vi "Leaderboard test 2.vi"() -> ()   [LabVIEW 2020, in "Visualisation.lvclass"]
uses:
  Visualisation.lvclass
  Application/Globals.vi
  Data Manager/Data Manager.lvclass
  Application/Application.lvlib
panel:
  out "Distance":T1(slide)={"Numeric"=0.0, "Numeric"=29.941887583444593, "Numeric"=34.779659813084116} scale=0.0..48.9661
  out "Leaderboard":T2(array[cluster]) {"Distance" scale=0.0..48.9661}
  out "B Total":dbl format="%0.1f km"
  out "A Total":dbl format="%0.1f km"
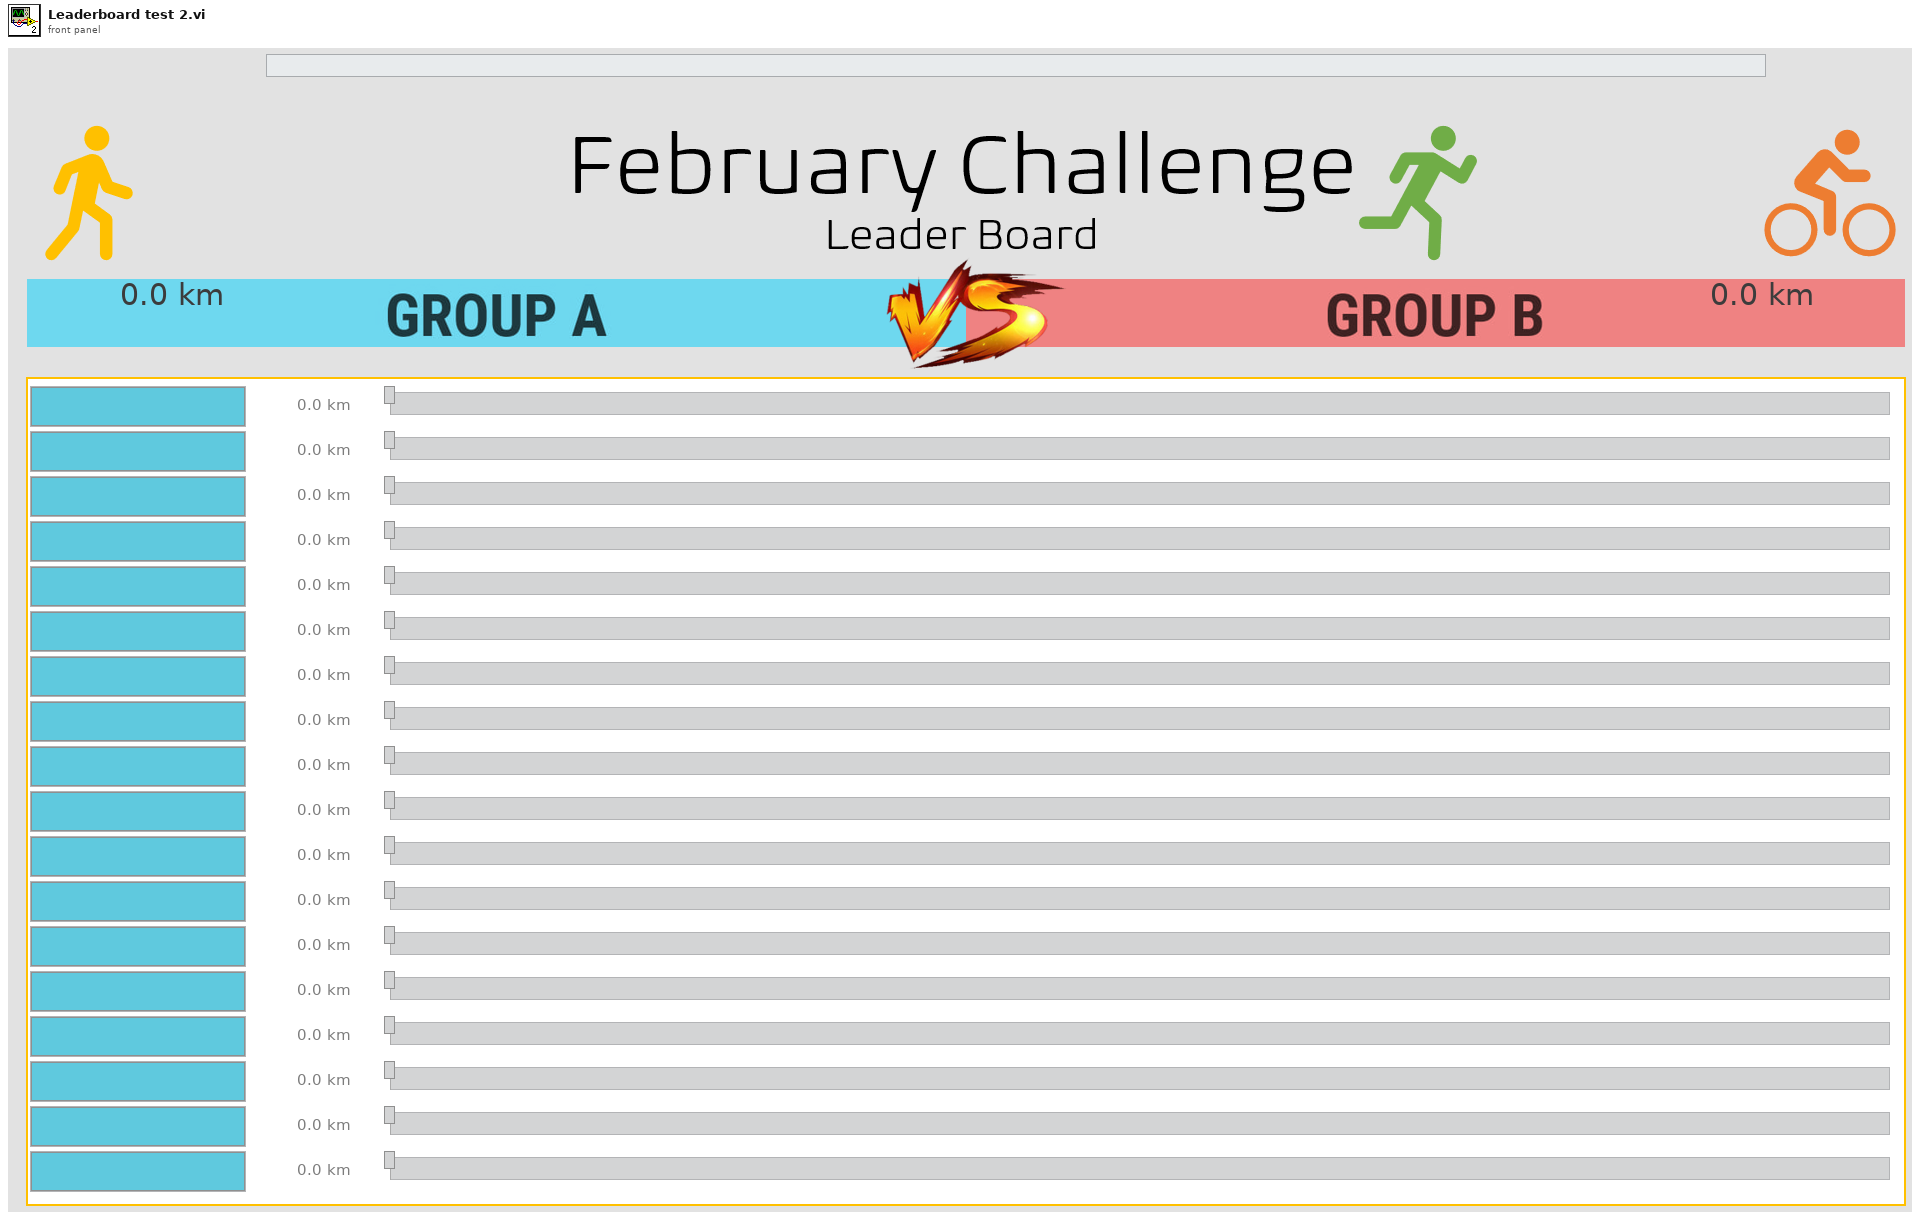
[diagram p1: front panel]
types:
  T1 = cluster{"Numeric":dbl, "Numeric":dbl, "Numeric":dbl}
  T2 = cluster{"Athlete":string, "Distance":dbl, "Team":u32}[]
  T3 = cluster{"Athlete":string, "Distance":dbl, "Team":u32}
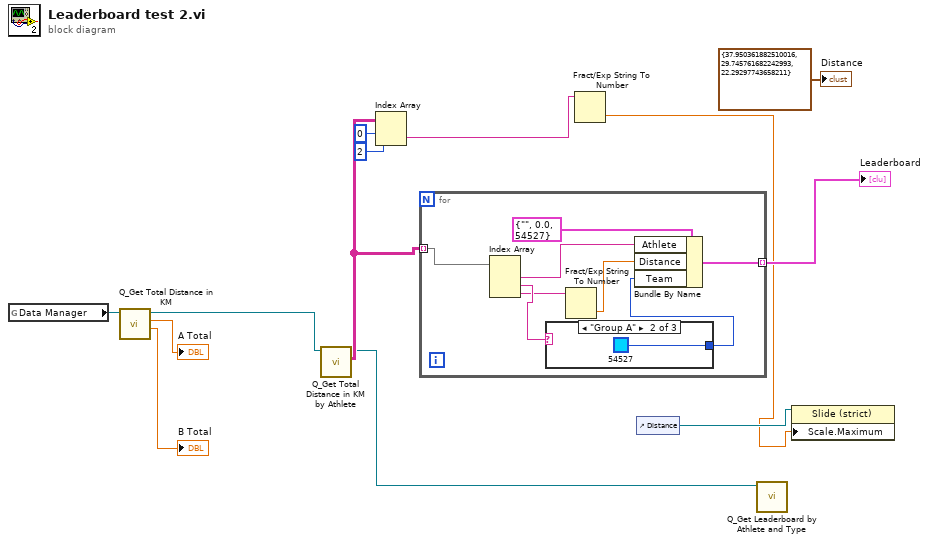
[diagram p0: block diagram]
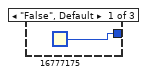
[diagram p2: hidden frame]
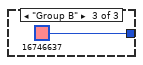
[diagram p3: hidden frame]
diagram:
  n1 = global read "Globals.vi" "Data Manager"() -> (w13:refnum<class "Data Manager.lvclass">)
  n2 = call-dynamic "Q_Get Total Distance in KM.vi"("Data Manager in"=w13) -> ("Group B"=→"B Total":dbl, "Group A"=→"A Total":dbl, "Data Manager out"=w10:refnum<class "Data Manager.lvclass">)  [unwired: 6 in, 2 out]
  n3 = call-dynamic "Q_Get Total Distance in KM by Athlete.vi"("Data Manager in"=w10) -> ("Result Set"=w3:string[][], "Data Manager out"=w1:refnum<class "Data Manager.lvclass">)  [unwired: 8 in, 1 out]
  n4 = Index Array(array=w3, index (row)=0, index (col)=2 ("disabled index (col)")) -> (element=w5:string)
  n5 = for {
    tunnel: w3 -> [w19] mode=indexing
    tunnel: [w20] -> w6 mode=indexing
    n6 = Index Array(array=w19) -> (element #1=w18:string, element #2=w15:string, element #3=w14:string)  [unwired: 3 in]
    n7 = case shown="\"Group A\"" w15 {
      tunnel: [u32 16777175 ("Color Box") u32 54527 ("Color Box") u32 16746637 ("Color Box")] -> w16
      frame "False", Default {
      }
      frame "Group A" {
      }
      frame "Group B" {
      }
    }
    n8 = Fract/Exp String To Number(string=w14) -> (number=w17:dbl)  [unwired: 3 in, 1 out]
    n9 = Bundle By Name(cluster=T3 {"Athlete"="", "Distance"=0.0, "Team"=54527} ("Leaderboard"), "Athlete"=w18, "Distance"=w17, "Team"=w16) -> (w20:T3)
  }
  "Leaderboard" <- w6
  n10 = Fract/Exp String To Number(string=w5) -> (number=w4:dbl)  [unwired: 3 in, 1 out]
  n11 = control-ref of="Distance"() -> (w9:refnum<vi>)
  n12 = call-dynamic "Q_Get Leaderboard by Athlete and Type.vi"("Data Manager in"=w1) -> ()  [unwired: 8 in, 3 out]
  n13 = property on="Property Node" class="Slide (strict)"(reference=w9, "Scale.Maximum"=w4) -> ()  [unwired: 1 in, 2 out]
  "Distance" <- T1 {"Numeric"=37.950361882510016, "Numeric"=29.745761682242993, "Numeric"=22.29297743658211} ("Distance")
